vi "Resize Listbox.vi"(7 "MulticolumnListbox in":refnum<vi>, 8 "error in (no error)":errorcluster, 9 "Column Offset [px] (47)":u32=47, 10 "Column Index (0)":i32, 11 "N Columns (3)":i32=3) -> (0 "error out":errorcluster)   [LabVIEW 2016]
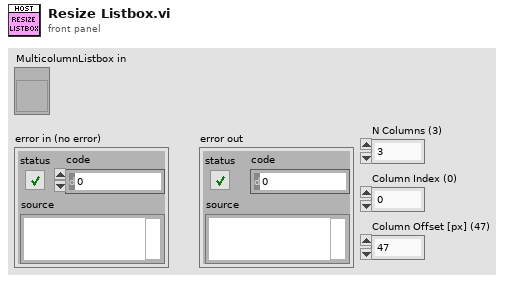
[diagram p1: front panel]
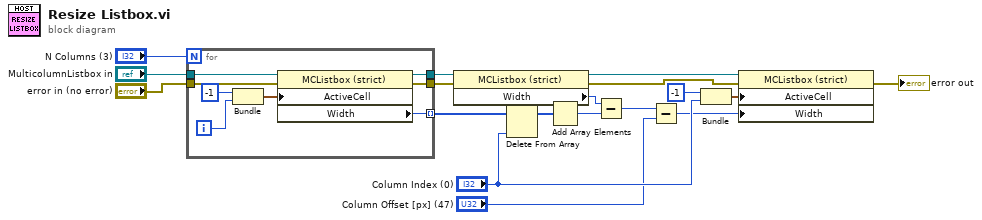
[diagram p0: block diagram]
diagram:
  n1 = for {
    N: "N Columns (3)" -> [_]
    tunnel: [w23] -> w15 mode=indexing
    tunnel: [w22] -> w16
    tunnel: "error in (no error)" -> [w21]
    tunnel: "MulticolumnListbox in" -> [w20]
    tunnel: [w19] -> w4
    i -> [w25]
    n2 = Bundle(-1, w25) -> (w26:cluster{i32, i32})  [unwired: 1 in]
    n3 = property on="Property Node" class="MCListbox (strict)"(reference=w20, error in=w21, "ActiveCell"=w26) -> (reference out=w19:refnum<vi>, error out=w22:errorcluster, "Width"=w23:u32)
  }
  n4 = property on="Property Node" class="MCListbox (strict)"(reference=w4, error in=w16) -> (reference out=w3:refnum<vi>, error out=w18:errorcluster, "Width"=w2:u32)
  n5 = Delete From Array(array=w15, index="Column Index (0)") -> (array with subset deleted=w14:u32[])  [unwired: 1 in, 1 out]
  n6 = Add Array Elements(numeric array=w14) -> (sum=w13:u32)
  n7 = Subtract(x=w2, y=w13) -> (x-y=w12:u32)
  n8 = Subtract(x=w12, y="Column Offset [px] (47)") -> (x-y=w8:u32)
  n9 = Bundle(-1, "Column Index (0)"="Column Index (0)") -> (w9:cluster{i32, "Column Index (0)":i32})  [unwired: 1 in]
  n10 = property on="Property Node" class="MCListbox (strict)"(reference=w3, error in=w18, "ActiveCell"=w9, "Width"=w8) -> (error out=→"error out":errorcluster)  [unwired: 1 out]
